vi "WedgeIntersectionGeometry.vi"(2 "rotate P to -y":bool, 3 "P":cluster{"x":dbl, "y":dbl, "z":dbl}={"x"=1.0, "y"=-3.0, "z"=1.0} {"x" format="%.2f"; "z" format="%.2f"; "y" format="%.2f"}, 4 "3D Parametric Surface":refnum<k7>(container), 5 "ct sphere":cluster{"radius":dbl, "theta":dbl, "phi":dbl}={"radius"=10.0, "theta"=160.0, "phi"=100.0} {"radius" format="%.2f"; "phi" format="%.2f"; "theta" format="%.2f"}, 6 "strip":cluster{"radius":dbl, "h":dbl, "a":dbl}={"radius"=4.0, "h"=1.0, "a"=3.0} {"radius" format="%.2f"; "a" format="%.2f"; "h" format="%.2f"}, 7 "Ring":i32(ring) items=["Spherical cap", "Center Strip", "Half Sphere", "Wedge"]) -> (1 "3D graph out":refnum<k7>)   [LabVIEW 2022 SP3]
uses:
  <vilib>/Platform/NI_3dgraph.lvlib
  <vilib>/gmath/NI_Gmath.lvlib
panel:
  in  "Case Constant\n(See Context Help) 2":bool
  in  "Case Constant\n(See Context Help)":bool
  out "error out":errorcluster
  out "Case Number":i32
  out "h(r,t) plot":dbl[](graph)
  in  "Save?":bool
  in  "scale factor":i32=4
  in  "planes":u16(ring) items=["test if r1 valid", "slice cap at h", "test if r5 valid"]
  out "distance":string[](array[string])
  out "Output Cluster":T1 {"r5" format="%.2f"; "r4" format="%.4f"; "r3" format="%.4f"; "r2" format="%.4f"; "r1" format="%.4f"; "r0" format="%.2f"}
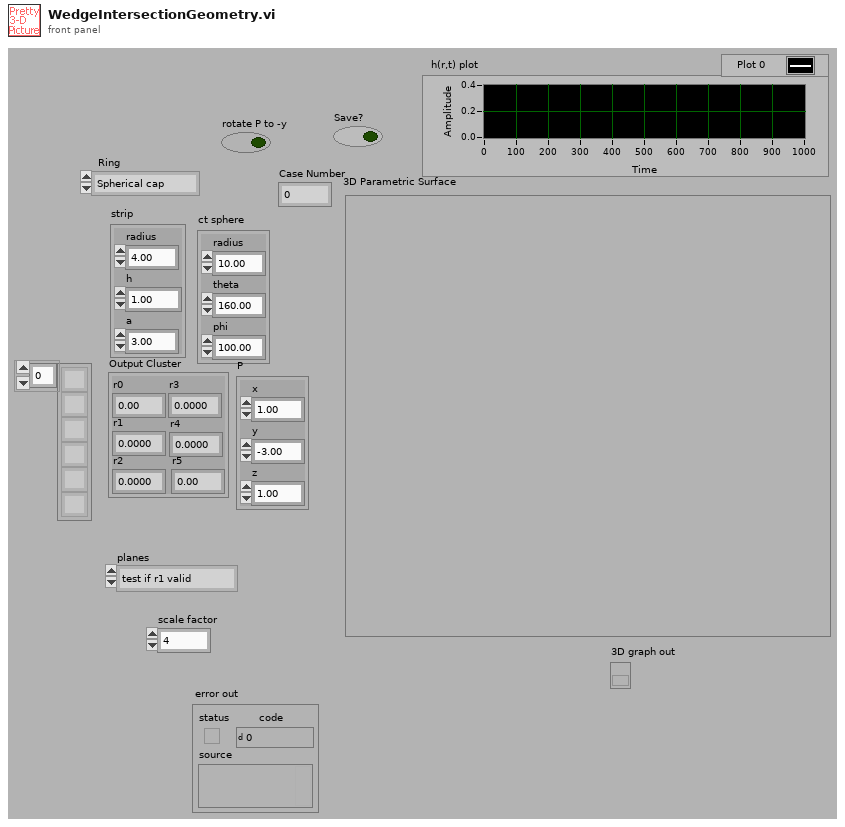
[diagram p1: front panel]
types:
  T1 = cluster{"r0":dbl, "r1":dbl, "r2":dbl, "r3":dbl, "r4":dbl, "r5":dbl}
  T2 = enum32{"existing file", "new file", "new or existing file", "existing dir", "new dir", "new or existing dir", "existing file (use LLBs)", "new file (use LLBs)", "new or existing file (use LLBs)", "new or existing file or directory (use LLBs)"}
  T3 = typedef "LVRectTypeDef.ctl" = cluster{"left":i16, "top":i16, "right":i16, "bottom":i16}
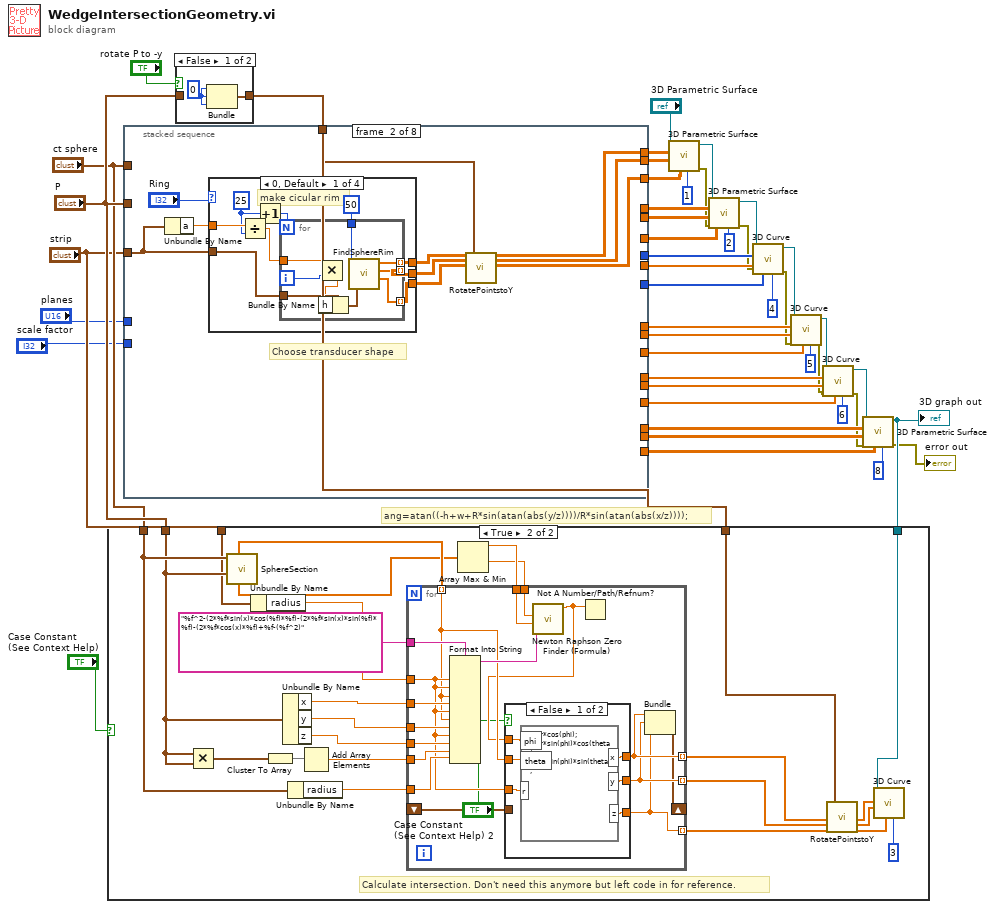
[diagram p0: block diagram]
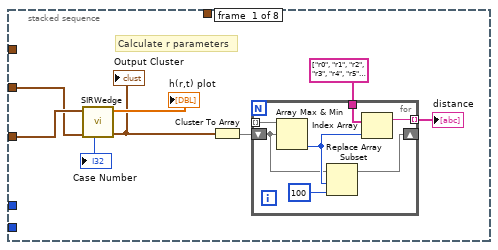
[diagram p2: hidden frame]
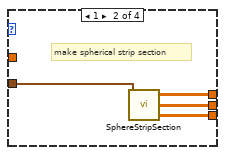
[diagram p3: hidden frame]
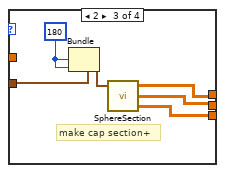
[diagram p4: hidden frame]
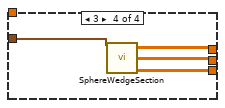
[diagram p5: hidden frame]
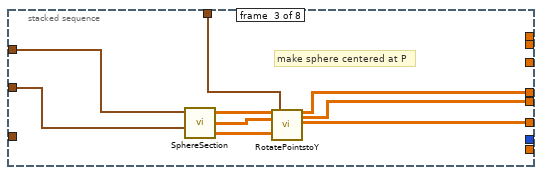
[diagram p6: hidden frame]
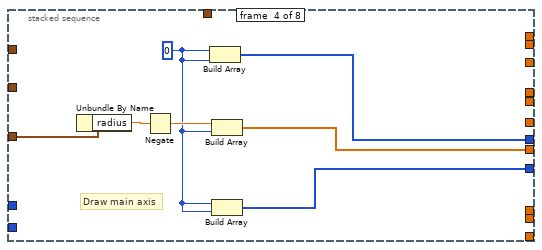
[diagram p7: hidden frame]
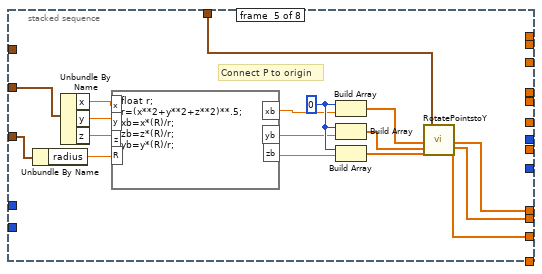
[diagram p8: hidden frame]
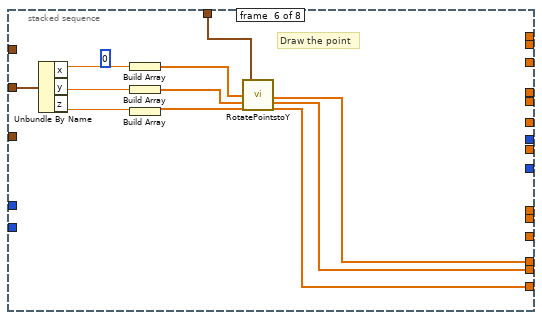
[diagram p9: hidden frame]
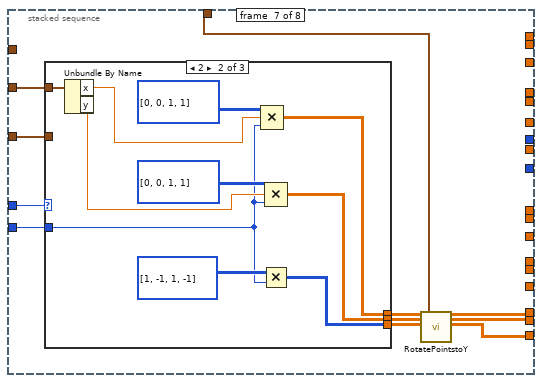
[diagram p10: hidden frame]
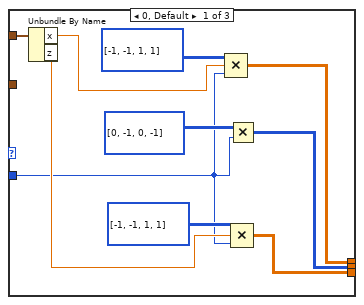
[diagram p11: hidden frame]
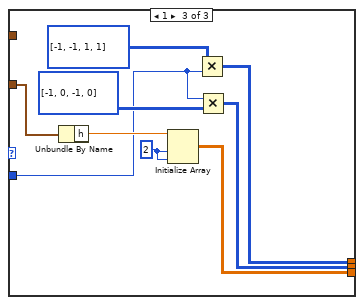
[diagram p12: hidden frame]
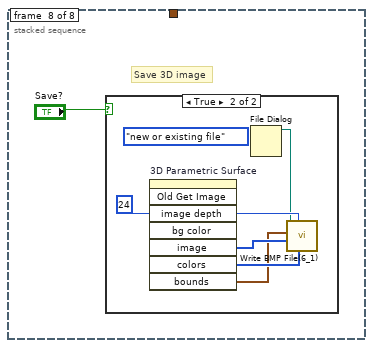
[diagram p13: hidden frame]
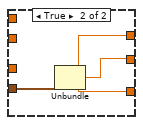
[diagram p16: hidden frame]
diagram:
  # "ang=atan((-h+w+R*sin(atan(abs(y/z))))/R*sin(atan(abs(x/z))));"
  n1 = case shown="False" "rotate P to -y" {
    tunnel: [w47 w48] -> w43
    tunnel: "P" -> [_ w48]
    frame False {
      w46 = 0
      n2 = Bundle(w46, w46, w46) -> (w47:cluster{i32, i32, i32})  [unwired: 1 out]
    }
    frame True {
    }
  }
  n3 = stacked-sequence {
    tunnel: "ct sphere" -> [_ _ w113 _ _ _ _ _]
    tunnel: "P" -> [w52 _ w109 _ w125 w141 w151 _]
    tunnel: w43 -> [_ w66 w108 _ w124 w142 w152 _]
    tunnel: "strip" -> [w53 w67 _ w120 w126 _ w159 _]
    tunnel: [_ w65 _ _ _ _ _ _] -> w39
    tunnel: [_ w64 _ _ _ _ _ _] -> w38
    tunnel: [_ w63 _ _ _ _ _ _] -> w37
    tunnel: [_ _ w107 _ _ _ _ _] -> w35
    tunnel: [_ _ w106 _ _ _ _ _] -> w34
    tunnel: [_ _ w105 _ _ _ _ _] -> w33
    tunnel: [_ _ _ w119 _ _ _ _] -> w31
    tunnel: [_ _ _ w118 _ _ _ _] -> w30
    tunnel: [_ _ _ w117 _ _ _ _] -> w29
    tunnel: [_ _ _ _ w123 _ _ _] -> w27
    tunnel: [_ _ _ _ w122 _ _ _] -> w26
    tunnel: [_ _ _ _ _ w140 _ _] -> w24
    tunnel: [_ _ _ _ _ w139 _ _] -> w23
    tunnel: [_ _ _ _ _ w138 _ _] -> w22
    tunnel: [_ _ _ _ w121 _ _ _] -> w15
    tunnel: [_ _ _ _ _ _ w153 _] -> w12
    tunnel: [_ _ _ _ _ _ w154 _] -> w11
    tunnel: [_ _ _ _ _ _ w155 _] -> w10
    tunnel: "planes" -> [_ _ _ _ _ _ w150 _]
    tunnel: "scale factor" -> [_ _ _ _ _ _ w149 _]
    frame #0 {
      # "Calculate r parameters"
      n4 = call "SIRWedge.vi"("P"=w52, "strip"=w53) -> ("r values (cm)"=w49:T1, "h wedge"=→"h(r,t) plot":dbl[], "Case Number"=→"Case Number":i32)  [unwired: 1 in, 6 out]
      "Output Cluster" <- w49
      n5 = Cluster To Array(cluster=w49) -> (array=w54:dbl[])
      n6 = for {
        tunnel: string[] ["r0", "r1", "r2", "r3", "r4", "r5", "r6", "r7", "r8"] ("Array Constant") -> [w59]
        tunnel: [w62] -> w55 mode=indexing
        shift-right: [w58] -> _
        shift-left: w54 -> [w57]
        tunnel: w54 -> [_] mode=indexing
        n7 = Array Max & Min(array=w57) -> (min index (indices)=w61:i32)  [unwired: 3 out]
        n8 = Replace Array Subset(array=w57, new element=100, index=w61) -> (w58:dbl[])
        n9 = Index Array(array=w59, index=w61) -> (element=w62:string)
      }
      "distance" <- w55
    }
    frame #1 {
      # "Choose transducer shape"
      n10 = Unbundle By Name(w67) -> ("a"=w72:dbl)
      n11 = case shown="0, Default" "Ring" {
        tunnel: [w80 w94 w100 w104] -> w71
        tunnel: [w79 w93 w99 w103] -> w70
        tunnel: [w78 w92 w98 w102] -> w69
        tunnel: w67 -> [w81 w91 w97 w101]
        tunnel: w72 -> [w77 _ _ _]
        frame 0, Default {
          w75 = 25
          # "make cicular rim"
          n12 = Divide(x=w77, y=w75) -> (x/y=w76:dbl)
          n13 = Increment(x=w75) -> (x+1=w73:i32)
          n14 = for {
            N: w73 -> [_]
            tunnel: w81 -> [w85]
            tunnel: [w90] -> w80 mode=indexing
            tunnel: [w89] -> w79 mode=indexing
            tunnel: [w88] -> w78 mode=indexing
            tunnel: w76 -> [w87]
            tunnel: 50 -> [w86]
            i -> [w82]
            n15 = Multiply(x=w87, y=w82) -> (x*y=w84:dbl)
            n16 = Bundle By Name(cluster=w85, "h"=w84) -> (w83:cluster{"radius":dbl, "h":dbl, "a":dbl})
            n17 = call "FindSphereRim.vi"("number of rim points"=w86, "strip (cm)"=w83) -> ("x"=w90:dbl[], "y"=w89:dbl[], "z"=w88:dbl[])  [unwired: 1 out]
          }
        }
        frame 1 {
          # "make spherical strip section"
          n18 = call "SphereStripSection.vi"("Ducer"=w91) -> ("x matrix"=w94:dbl[][], "y matrix"=w93:dbl[][], "z matrix"=w92:dbl[][])  [unwired: 1 in, 4 out]
        }
        frame 2 {
          w95 = 180
          # "make cap section+"
          n19 = Bundle(cluster=w97, "h"=w95, "a"=w95) -> (w96:cluster{"radius":dbl, "h":dbl, "a":dbl})  [unwired: 1 out]
          n20 = call "SphereSection.vi"("Ducer"=w96) -> ("x matrix"=w100:dbl[][], "y matrix"=w99:dbl[][], "z matrix"=w98:dbl[][])  [unwired: 2 in, 3 out]
        }
        frame 3 {
          n21 = call "SphereWedgeSection.vi"("Ducer"=w101) -> ("x matrix"=w104:dbl[][], "y matrix"=w103:dbl[][], "z matrix"=w102:dbl[][])  [unwired: 1 in, 4 out]
        }
      }
      n22 = call "RotatePointstoY.vi"("x matrix"=w71, "y matrix"=w70, "z matrix"=w69, "P"=w66) -> ("x matrix"=w65:dbl[][], "y matrix"=w64:dbl[][], "z matrix"=w63:dbl[][])  [unwired: 3 in, 10 out]
    }
    frame #2 {
      # "make sphere centered at P"
      n23 = call "SphereSection.vi"("Ducer"=w113, "P"=w109) -> ("x matrix"=w112:dbl[][], "y matrix"=w111:dbl[][], "z matrix"=w110:dbl[][])  [unwired: 1 in, 3 out]
      n24 = call "RotatePointstoY.vi"("x matrix"=w112, "y matrix"=w111, "z matrix"=w110, "P"=w108) -> ("x matrix"=w107:dbl[][], "y matrix"=w106:dbl[][], "z matrix"=w105:dbl[][])  [unwired: 3 in, 10 out]
    }
    frame #3 {
      w115 = 0
      # "Draw main axis"
      n25 = Unbundle By Name(w120) -> ("radius"=w114:dbl)
      n26 = Negate(x=w114) -> (-x=w116:dbl)
      n27 = Build Array(w115, w115) -> (w119:i32[])
      n28 = Build Array(w116, w115) -> (w118:dbl[])
      n29 = Build Array(w115, w115) -> (w117:i32[])
    }
    frame #4 {
      w137 = 0
      # "Connect P to origin"
      n30 = Unbundle By Name(w126) -> ("radius"=w127:dbl)
      n31 = Unbundle By Name(w125) -> ("x"=w130:dbl, "y"=w129:dbl, "z"=w128:dbl)
      n32 = formula code="float r;\nr=(x**2+y**2+z**2)**.5;\nxb=x*(R)/r;\nzb=z*(R)/r;\nyb=y*(R)/r;"("z"=w128, "x"=w130, "y"=w129, "R"=w127) -> ("xb"=w131:dbl, "yb"=w136:dbl, "zb"=w135:dbl)
      n33 = Build Array(w137, w131) -> (w133:dbl[])
      n34 = Build Array(w137, w136) -> (w134:dbl[])
      n35 = Build Array(w137, w135) -> (w132:dbl[])
      n36 = call "RotatePointstoY.vi"("x matrix 1D"=w133, "y matrix 1D"=w134, "z matrix 1D"=w132, "P"=w124) -> ("x matrix1D"=w123:dbl[], "y matrix 1D"=w122:dbl[], "z matrix 1D"=w121:dbl[])  [unwired: 3 in, 10 out]
    }
    frame #5 {
      (unwired) 0
      # "Draw the point"
      n37 = Unbundle By Name(w141) -> ("x"=w148:dbl, "y"=w147:dbl, "z"=w146:dbl)
      n38 = Build Array(w148) -> (w143:dbl[])
      n39 = Build Array(w147) -> (w145:dbl[])
      n40 = Build Array(w146) -> (w144:dbl[])
      n41 = call "RotatePointstoY.vi"("x matrix 1D"=w143, "y matrix 1D"=w145, "z matrix 1D"=w144, "P"=w142) -> ("x matrix1D"=w140:dbl[], "y matrix 1D"=w139:dbl[], "z matrix 1D"=w138:dbl[])  [unwired: 3 in, 10 out]
    }
    frame #6 {
      n42 = case shown="2" w150 {
        tunnel: w159 -> [_ _ w185]
        tunnel: [w163 w173 w183] -> w158
        tunnel: [w162 w171 w182] -> w157
        tunnel: [w161 w172 w181] -> w156
        tunnel: w151 -> [w169 w179 _]
        tunnel: w149 -> [w160 w170 w180]
        frame 0, Default {
          n43 = Unbundle By Name(w169) -> ("x"=w167:dbl, "z"=w165:dbl)
          n44 = Compound Arithmetic op=MULTIPLY(i32[][] [[-1, -1], [1, 1]], w167, w160) -> (w163:dbl[][])
          n45 = Multiply(x=i32[][] [[0, -1], [0, -1]], y=w160) -> (x*y=w162:i32[][])
          n46 = Compound Arithmetic op=MULTIPLY(i32[][] [[-1, -1], [1, 1]], w165, w160) -> (w161:dbl[][])
        }
        frame 2 {
          n47 = Unbundle By Name(w179) -> ("x"=w177:dbl, "y"=w175:dbl)
          n48 = Compound Arithmetic op=MULTIPLY(i32[][] [[0, 0], [1, 1]], w177, w170) -> (w173:dbl[][])
          n49 = Multiply(x=i32[][] [[1, -1], [1, -1]], y=w170) -> (x*y=w172:i32[][])
          n50 = Compound Arithmetic op=MULTIPLY(i32[][] [[0, 0], [1, 1]], w175, w170) -> (w171:dbl[][])
        }
        frame 1 {
          w188 = 2
          n51 = Unbundle By Name(w185) -> ("h"=w184:dbl)
          n52 = Initialize Array(w184, w188, w188) -> (w181:dbl[][])
          n53 = Multiply(x=i32[][] [[-1, -1], [1, 1]], y=w180) -> (x*y=w183:i32[][])
          n54 = Multiply(x=w180, y=i32[][] [[-1, 0], [-1, 0]]) -> (x*y=w182:i32[][])
        }
      }
      n55 = call "RotatePointstoY.vi"("x matrix"=w158, "y matrix"=w157, "z matrix"=w156, "P"=w152) -> ("x matrix"=w155:dbl[][], "y matrix"=w154:dbl[][], "z matrix"=w153:dbl[][])  [unwired: 3 in, 10 out]
    }
    frame #7 {
      # "Save 3D image"
      n56 = case shown="True" "Save?" {
        frame False {
        }
        frame True {
          (unwired) T2."new or existing file" ("select mode (2)")
          w194 = 24
          n57 = invoke on="3D Parametric Surface" class="AXCont" method="Old Get Image"("image depth"=w194) -> ("image"=w192:u8[], "colors"=w193:u32[], "bounds"=w191:T3)  [unwired: 7 in, 5 out]
          n58 = File Dialog() -> (3:w190:path)  [unwired: 1 in, 9 out]
          n59 = call <vilib>:"Write BMP File(6_1).vi"("color table"=w193, "depth"=w194, "flattened image data"=w192, "rect"=w191, "path to BMP file"=w190) -> ()  [unwired: 1 in, 6 out]
        }
      }
    }
  }
  n60 = call <vilib>:"3D Parametric Surface.vi"("plot number (1)"=1, "z matrix"=w37, "y matrix"=w38, "x matrix"=w39, "3D graph"="3D Parametric Surface") -> ("error out"=w6:errorcluster, "3D graph out"=w19:refnum<k7>)  [unwired: 1 in, 4 out]
  n61 = call <vilib>:"3D Parametric Surface.vi"("plot number (1)"=2, "z matrix"=w33, "error in (no error)"=w6, "y matrix"=w34, "x matrix"=w35, "3D graph"=w19) -> ("error out"=w5:errorcluster, "3D graph out"=w18:refnum<k7>)  [unwired: 4 out]
  n62 = call <vilib>:"3D Curve.vi"("plot number (1)"=4, "z vector"=w29, "error in (no error)"=w5, "y vector"=w30, "x vector"=w31, "3D graph"=w18) -> ("error out"=w4:errorcluster, "3D graph out"=w17:refnum<k7>)  [unwired: 4 out]
  n63 = call <vilib>:"3D Curve.vi"("plot number (1)"=5, "z vector"=w15, "error in (no error)"=w4, "y vector"=w26, "x vector"=w27, "3D graph"=w17) -> ("error out"=w3:errorcluster, "3D graph out"=w16:refnum<k7>)  [unwired: 4 out]
  n64 = call <vilib>:"3D Curve.vi"("plot number (1)"=6, "z vector"=w22, "error in (no error)"=w3, "y vector"=w23, "x vector"=w24, "3D graph"=w16) -> ("error out"=w2:errorcluster, "3D graph out"=w14:refnum<k7>)  [unwired: 4 out]
  n65 = call <vilib>:"3D Parametric Surface.vi"("plot number (1)"=8, "z matrix"=w12, "error in (no error)"=w2, "y matrix"=w11, "x matrix"=w10, "3D graph"=w14) -> ("error out"=→"error out":errorcluster, "3D graph out"=w9:refnum<k7>)  [unwired: 4 out]
  "3D graph out" <- w9
  n66 = case shown="True" "Case Constant\n(See Context Help)" {
    tunnel: "ct sphere" -> [_ w201]
    tunnel: "P" -> [_ w200]
    tunnel: w43 -> [_ w202]
    tunnel: "strip" -> [_ w197]
    tunnel: w9 -> [_ w195]
    frame False {
    }
    frame True {
      # "Calculate intersection. Don't need this anymore but left code in for reference."
      n67 = Multiply(x=w200, y=w200) -> (x*y=w219:cluster{"x":dbl, "y":dbl, "z":dbl})
      n68 = call "SphereSection.vi"("Ducer"=w201, "P"=w200) -> ("thetas"=w199:dbl[], "phis"=w198:dbl[])  [unwired: 1 in, 4 out]
      n69 = Unbundle By Name(w197) -> ("radius"=w196:dbl)
      n70 = Cluster To Array(cluster=w219) -> (array=w218:dbl[])
      n71 = Unbundle By Name(w200) -> ("x"=w210:dbl, "y"=w211:dbl, "z"=w209:dbl)
      n72 = Unbundle By Name(w201) -> ("radius"=w215:dbl)
      n73 = Add Array Elements(numeric array=w218) -> (sum=w216:dbl)
      n74 = Array Max & Min(array=w198) -> (max value=w213:dbl, min value=w212:dbl)  [unwired: 2 out]
      n75 = for {
        tunnel: "%f^2-(2*%f*sin(x)*cos(%f)*%f)-(2*%f*sin(x)*sin(%f)*%f)-(2*%f*cos(x)*%f)+%f-(%f^2)" ("formula") -> [w230]
        tunnel: w210 -> [w237]
        tunnel: w211 -> [w236]
        tunnel: w196 -> [w228]
        tunnel: w209 -> [w235]
        tunnel: w216 -> [w234]
        tunnel: w215 -> [w233]
        tunnel: w199 -> [w227] mode=indexing
        tunnel: [w226] -> w203 mode=indexing
        tunnel: [w225] -> w204 mode=indexing
        tunnel: [w224] -> w205 mode=indexing
        tunnel: w213 -> [w232]
        tunnel: w212 -> [w231]
        shift-right: [w223] -> _
        shift-left: _ -> [w222]
        n76 = Format Into String(format string=w230, w228, w228, w227, w237, w228, w227, w236, w228, w235, w234, w233) -> (resulting string=w229:string)  [unwired: 2 in, 1 out]
        n77 = call <vilib>:"Newton Raphson Zero Finder (Formula).vi"("formula"=w229, "end"=w232, "start"=w231) -> ("zero"=w221:dbl)  [unwired: 5 in, 3 out]
        n78 = case shown="False" "Case Constant\n(See Context Help) 2" {
          tunnel: [w243 w246] -> w226
          tunnel: [w242 w245] -> w225
          tunnel: [w241 w244] -> w224
          tunnel: w228 -> [w240 _]
          tunnel: w227 -> [w239 _]
          tunnel: w222 -> [_ w247]
          tunnel: w221 -> [w238 _]
          frame False {
            n79 = formula code="z=r*cos(phi);\nx=r*sin(phi)*cos(theta);\ny=r*sin(phi)*sin(theta);"("r"=w240, "phi"=w238, "theta"=w239) -> ("x"=w243:dbl, "y"=w242:dbl, "z"=w241:dbl)
          }
          frame True {
            n80 = Unbundle(w247) -> ("x"=w246:dbl, "y"=w245:dbl, "z"=w244:dbl)
          }
        }
        n81 = Not A Number/Path/Refnum?(number/path/refnum=w221) -> ()  [unwired: 1 out]
        n82 = Bundle("x"=w226, "y"=w225, "z"=w224) -> (w223:cluster{"x":dbl, "y":dbl, "z":dbl})  [unwired: 1 out]
      }
      n83 = call "RotatePointstoY.vi"("x matrix 1D"=w203, "y matrix 1D"=w204, "z matrix 1D"=w205, "P"=w202) -> ("x matrix1D"=w207:dbl[], "y matrix 1D"=w206:dbl[], "z matrix 1D"=w208:dbl[])  [unwired: 3 in, 10 out]
      n84 = call <vilib>:"3D Curve.vi"("plot number (1)"=3, "z vector"=w208, "y vector"=w206, "x vector"=w207, "3D graph"=w195) -> ()  [unwired: 1 in, 6 out]
    }
  }
